vi "写入baud rate.vi"(8 "error in (no error)":errorcluster caption="错误输入（无错误）", 10 "baud rate":u32=9600 caption="波特率(9600)", 11 "串口配置输入":refnum<class "串口配置.lvclass">) -> (0 "error out":errorcluster caption="错误输出", 3 "串口配置输出":refnum<class "串口配置.lvclass">)   [LabVIEW 2013, in "串口配置.lvclass"]
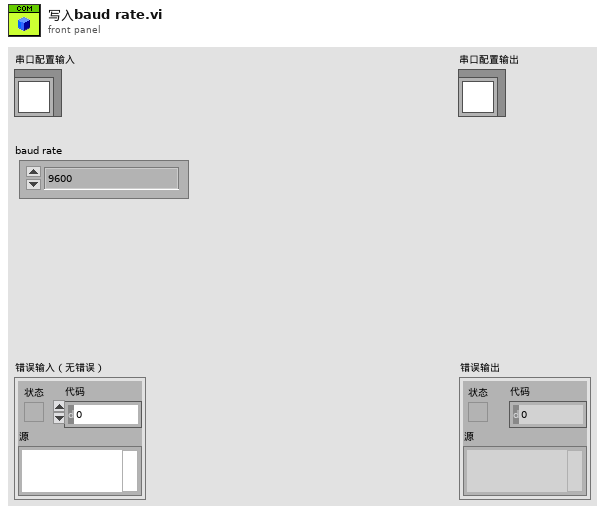
[diagram p1: front panel]
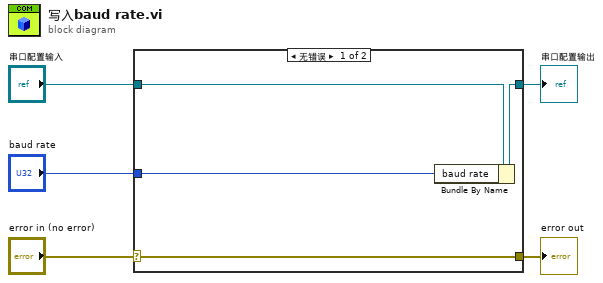
[diagram p0: block diagram]
diagram:
  n1 = case shown="无错误" "error in (no error)" {
    selector: "error in (no error)" -> [w9 w10]
    tunnel: [w9 w10] -> w4
    tunnel: [w7 w11] -> w2
    tunnel: "串口配置输入" -> [w8 w11]
    tunnel: "baud rate" -> [w6 _]
    frame No Error {
      n2 = Bundle By Name(cluster=w8, "baud rate"=w6) -> (w7:refnum<class "串口配置.lvclass">)
    }
    frame Error {
    }
  }
  "error out" <- w4
  "串口配置输出" <- w2
